vi "write_ui_elements.vi"(8 "error in (no error)":errorcluster, 10 "ui_elements":T1, 11 "panel in":refnum<class "panel.lvclass">) -> (0 "error out":errorcluster, 3 "panel out":refnum<class "panel.lvclass">)   [LabVIEW 2015, in "panel.lvclass"]
uses:
  panel.lvclass
  ui_elements.ctl
  panel.lvclass/panel.ctl
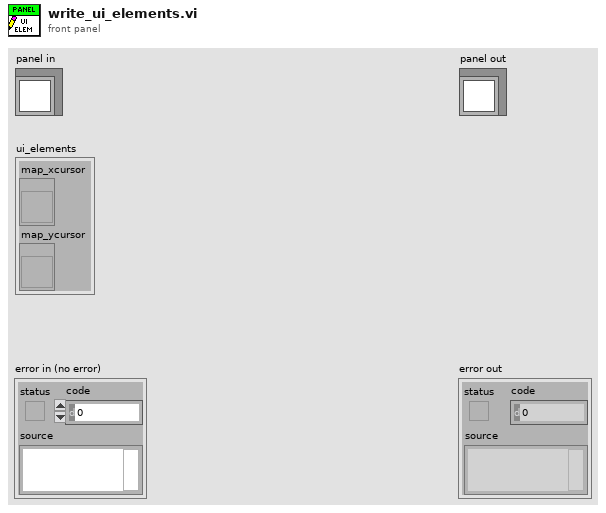
[diagram p1: front panel]
types:
  T1 = typedef "ui_elements.ctl" = cluster{"map_xcursor":refnum<vi>, "map_ycursor":refnum<vi>}
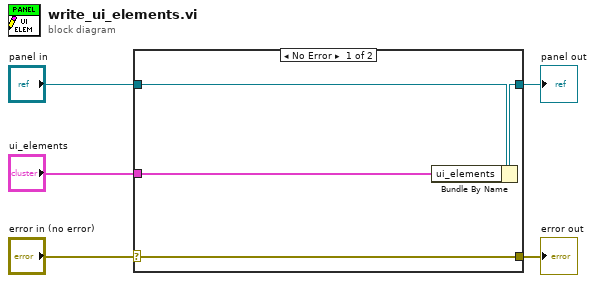
[diagram p0: block diagram]
diagram:
  n1 = case shown="No Error" "error in (no error)" {
    selector: "error in (no error)" -> [w9 w10]
    tunnel: [w9 w10] -> w4
    tunnel: [w7 w11] -> w2
    tunnel: "panel in" -> [w8 w11]
    tunnel: "ui_elements" -> [w6 _]
    frame No Error {
      n2 = Bundle By Name(cluster=w8, "ui_elements"=w6) -> (w7:refnum<class "panel.lvclass">)
    }
    frame Error {
    }
  }
  "error out" <- w4
  "panel out" <- w2
